vi "AWS-S3-ProgressCallbackUpload.vi"(4 "Initial Params":T1, 5 "Event Data":cluster{"sender":refnum<k24>, "e":refnum<k24>}, 6 "Control Ref":refnum<k24>, 7 "Event Common Data":T2) -> ()   [LabVIEW 2012, in "AWS-S3-API.lvclass"]
uses:
  AWS-S3-API.lvclass
  C:/Users/Jack/repo/aws/AWS-SDK/AWSSDK.dll
  repo/aws/AWS-SDK/AWSSDK.dll
  AWS-S3-Transfer-Progress.ctl
  AWS-S3-Transfer-Header.ctl
panel:
  # "Inputs"
  # "Outputs"
  # "No Outputs - this VI\nis fire and forget"
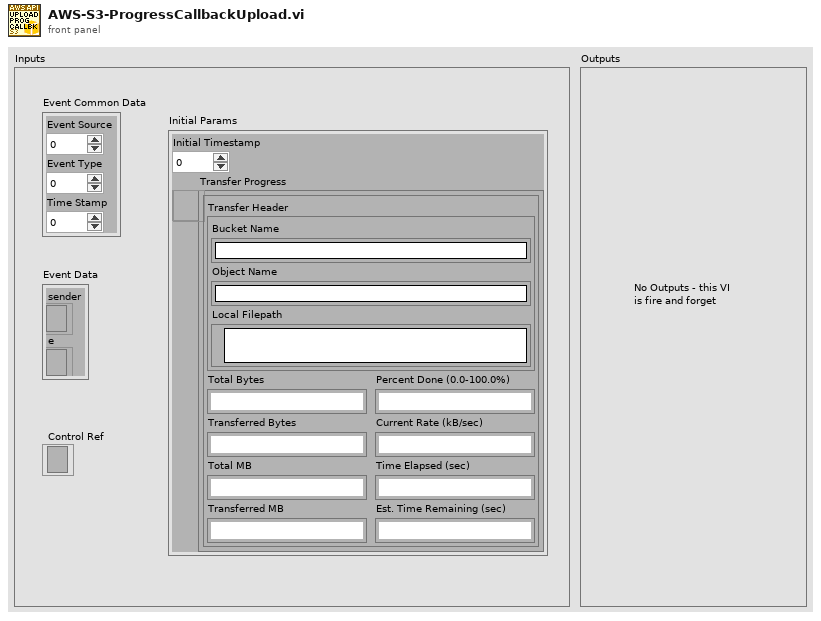
[diagram p1: front panel]
types:
  T1 = cluster{"Initial Timestamp":u32, "Transfer Progress":refnum<user-event>}
  T2 = cluster{"Event Source":i32, "Event Type":u32, "Time Stamp":u32}
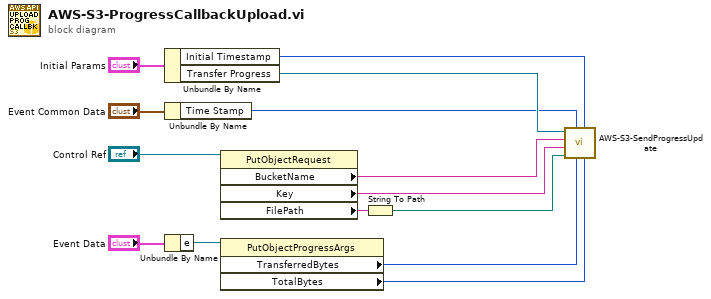
[diagram p0: block diagram]
diagram:
  n1 = Unbundle By Name("Initial Params") -> ("Initial Timestamp"=w8:u32, "Transfer Progress"=w9:refnum<user-event>)
  n2 = Unbundle By Name("Event Common Data") -> ("Time Stamp"=w7:u32)
  n3 = Unbundle By Name("Event Data") -> ("e"=w13:refnum<k24>)
  n4 = property class="PutObjectRequest"(reference="Control Ref") -> ("BucketName"=w6:string, "Key"=w5:string, "FilePath"=w4:string)  [unwired: 1 in, 2 out]
  n5 = property class="PutObjectProgressArgs"(reference=w13) -> ("TransferredBytes"=w2:i64, "TotalBytes"=w1:i64)  [unwired: 1 in, 2 out]
  n6 = String To Path(string=w4) -> (path=w3:path)
  n7 = call "AWS-S3-SendProgressUpdate.vi"("TotalBytes"=w1, "Initial Timestamp"=w8, "TransferredBytes"=w2, "Time Stamp"=w7, "Local Filepath"=w3, "Key"=w5, "BucketName"=w6, "User Event in"=w9) -> ()  [unwired: 4 in]
